vi "repPrepareGoalKickAllyPlayVSS.vi"(8 "error in (no error)":errorcluster, 11 "PrepareGoalKickAllyPlayVSS in":refnum<class "PrepareGoalKickAllyPlayVSS.lvclass">) -> (0 "error out":errorcluster, 3 "PrepareGoalKickAllyPlayVSS out":refnum<class "PrepareGoalKickAllyPlayVSS.lvclass">)   [LabVIEW 2020, in "PrepareGoalKickAllyPlayVSS.lvclass"]
uses:
  PrepareGoalKickAllyPlayVSS.lvclass
  Field_class/Field.lvclass
  Game_class/Game.lvclass
panel:
  out "RobotPlacement 2":T1(array[cluster])
  in  "Game in 2":refnum<class "Game.lvclass">
  in  "RobotPlacement":T1(array[cluster])
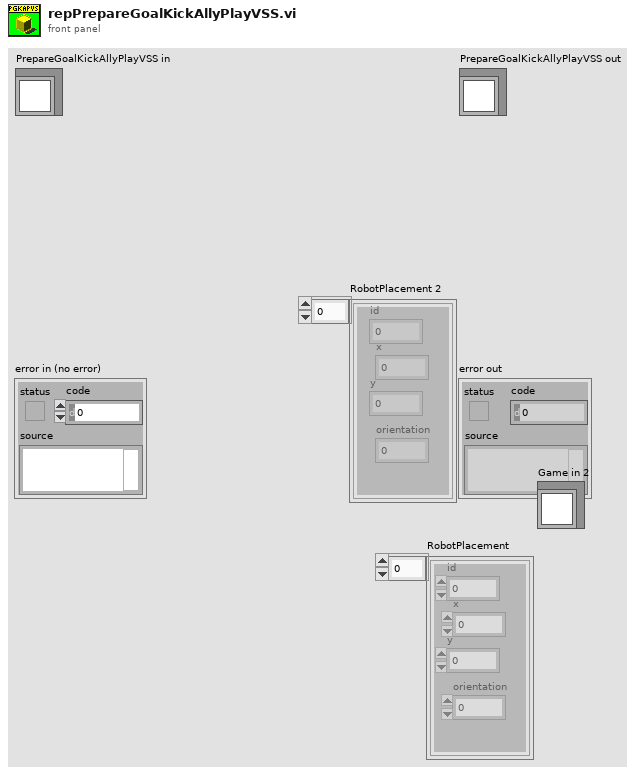
[diagram p1: front panel]
types:
  T1 = cluster{"id":i32, "x":dbl, "y":dbl, "orientation":dbl}[]
  T2 = cluster{"id":i32, "x":dbl, "y":dbl, "orientation":dbl}
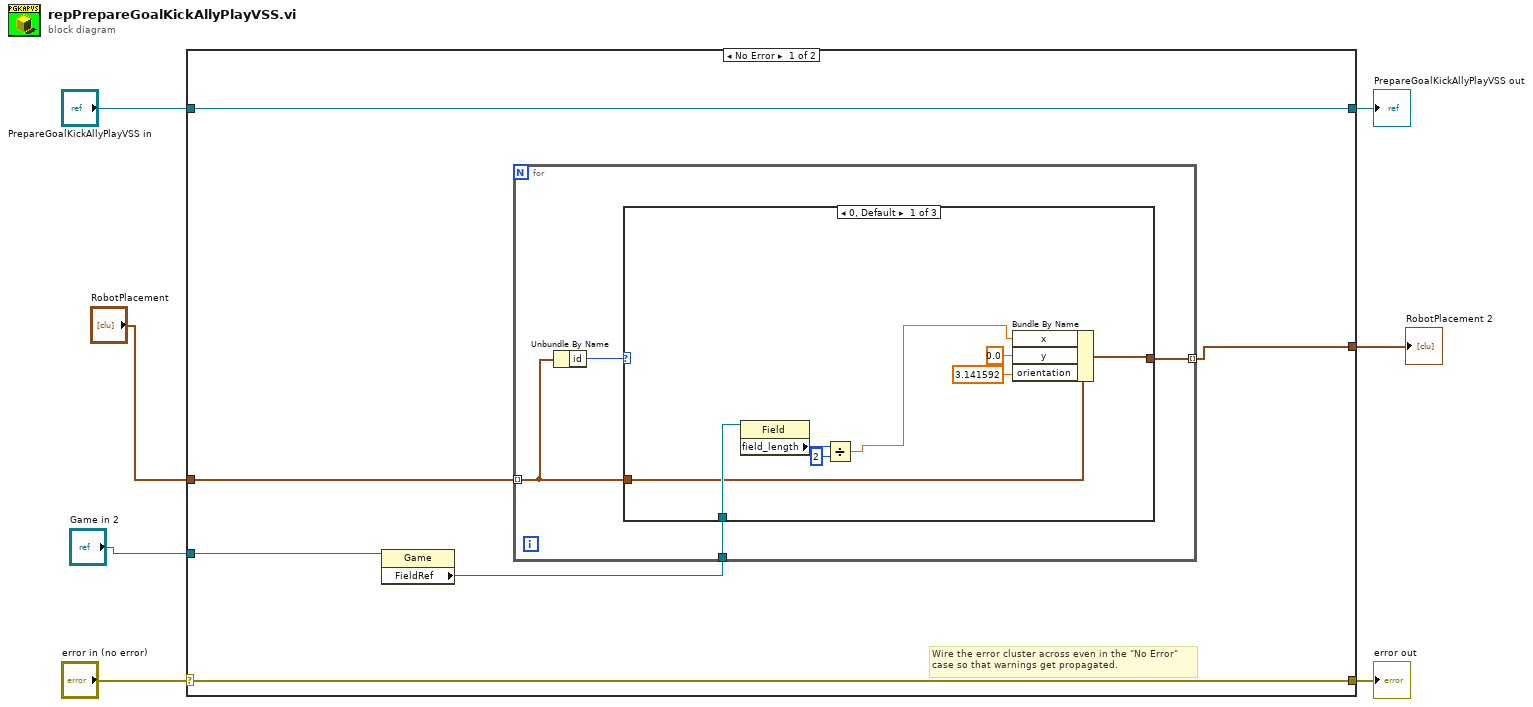
[diagram p0: block diagram]
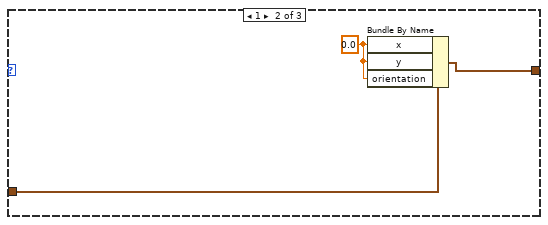
[diagram p2: hidden frame]
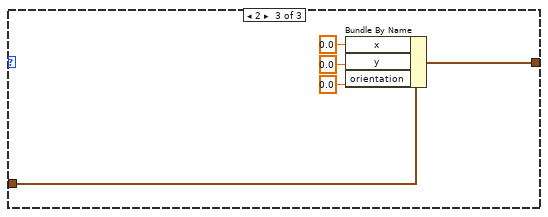
[diagram p3: hidden frame]
diagram:
  n1 = case shown="No Error" "error in (no error)" {
    selector: "error in (no error)" -> [w12 w35]
    tunnel: [w12 w35] -> w6
    tunnel: [w13 w34] -> w4
    tunnel: "PrepareGoalKickAllyPlayVSS in" -> [w13 w34]
    tunnel: [w10 _] -> w3
    tunnel: "RobotPlacement" -> [w9 _]
    tunnel: "Game in 2" -> [w8 _]
    frame No Error {
      # "Wire the error cluster across even in the \"No Error\"\ncase so that warnings get propagated."
      n2 = property class="Game"(reference=w8) -> ("FieldRef"=w11:refnum<class "Field.lvclass">)  [unwired: 1 in, 2 out]
      n3 = for {
        tunnel: [w17] -> w10 mode=indexing
        tunnel: w11 -> [w16]
        tunnel: w9 -> [w14] mode=indexing
        n4 = Unbundle By Name(w14) -> ("id"=w15:i32)
        n5 = case shown="0, Default" w15 {
          tunnel: [w25 w27 w33] -> w17
          tunnel: w16 -> [w24 _ _]
          tunnel: w14 -> [w18 w26 w29]
          frame 0, Default {
            n6 = property class="Field"(reference=w24) -> ("field_length"=w23:i32)  [unwired: 1 in, 2 out]
            n7 = Divide(x=w23, y=2) -> (x/y=w21:dbl)
            n8 = Bundle By Name(cluster=w18, "x"=w21, "y"=0.0, "orientation"=3.141592) -> (w25:T2)
          }
          frame 1 {
            w28 = 0.0 ("x")
            n9 = Bundle By Name(cluster=w26, "x"=w28, "y"=w28, "orientation"=w28) -> (w27:T2)
          }
          frame 2 {
            n10 = Bundle By Name(cluster=w29, "x"=0.0, "y"=0.0, "orientation"=0.0) -> (w33:T2)
          }
        }
      }
    }
    frame Error {
    }
  }
  "error out" <- w6
  "PrepareGoalKickAllyPlayVSS out" <- w4
  "RobotPlacement 2" <- w3
